vi "Write Var_Indexes.vi"(8 "error in (no error)":errorcluster, 10 "Var_Indexes":refnum<class "Var_Index.lvclass">[](array[class]), 11 "Var_Access in":refnum<class "Var_Access.lvclass">) -> (0 "error out":errorcluster, 3 "Var_Access out":refnum<class "Var_Access.lvclass">)   [LabVIEW 2021, in "Var_Access.lvclass"]
uses:
  Var_Access.lvclass
  Var Index/Var_Index.lvclass
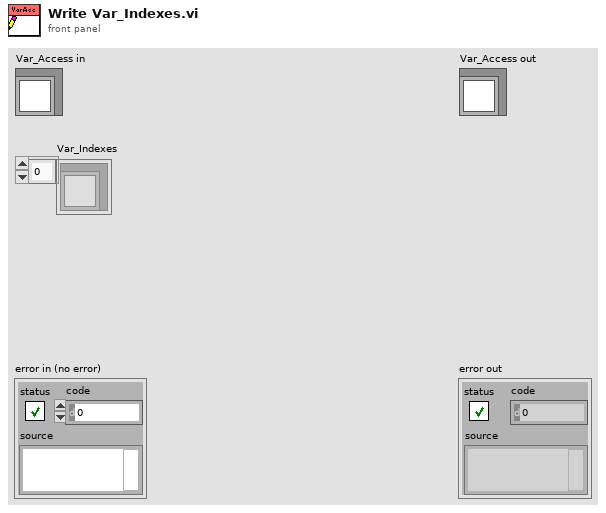
[diagram p1: front panel]
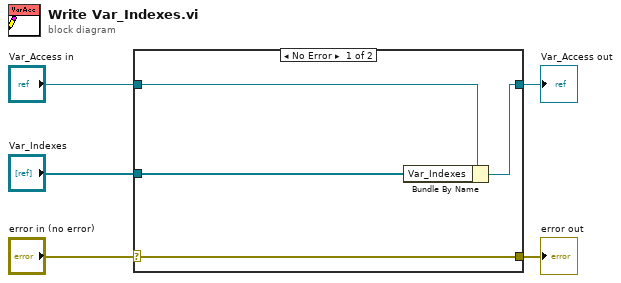
[diagram p0: block diagram]
diagram:
  n1 = case shown="No Error" "error in (no error)" {
    selector: "error in (no error)" -> [w9 w10]
    tunnel: [w9 w10] -> w4
    tunnel: [w7 w11] -> w2
    tunnel: "Var_Access in" -> [w8 w11]
    tunnel: "Var_Indexes" -> [w6 _]
    frame No Error {
      n2 = Bundle By Name(cluster=w8, "Var_Indexes"=w6) -> (w7:refnum<class "Var_Access.lvclass">)
    }
    frame Error {
    }
  }
  "error out" <- w4
  "Var_Access out" <- w2
